vi "GetSetRegister.vi"(7 "Set?":bool, 8 "error in (no error)":errorcluster, 9 "Bytes in":string, 10 "Register Name":string, 11 "Camera in":refnum<class "Camera.lvclass">) -> (0 "error out":errorcluster, 1 "Bytes out":string)   [LabVIEW 2020, in "Camera.lvclass"]
uses:
  Camera.lvclass
  Camera.lvclass/Camera.ctl
  bin/gindustrialcam_32-1.dll
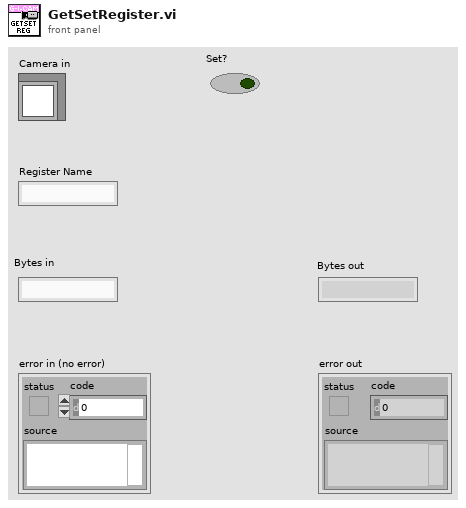
[diagram p1: front panel]
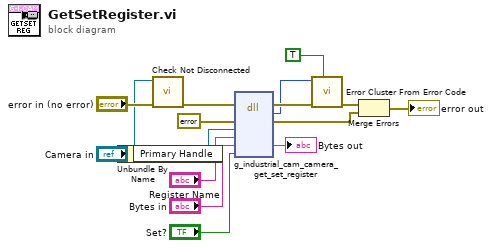
[diagram p0: block diagram]
diagram:
  n1 = Unbundle By Name("Camera in") -> ("Primary Handle"=w5:refnum<data-value>)
  n2 = call "Check Not Disconnected.vi"("error in (no error)"="error in (no error)", "Camera in"="Camera in") -> ("error out"=w2:errorcluster)  [unwired: 9 in]
  n3 = dll-call lib="C:/serenial/lib/g-industrial-camera/LabVIEW/g_industrial_cam/bin/gindustrialcam_*-1.*" fn="g_industrial_cam_camera_get_set_register"(error in=w2, "err"=errorcluster {"status"=FALSE, "code"=0, "source"=""} ("error constant"), "edvr"=w5, "name"="Register Name", "value"="Bytes in", "set"="Set?") -> (error out=w15:errorcluster, "Mg_Error"=w14:i32, "err"=w12:errorcluster, "value"=→"Bytes out":string)  [unwired: 5 in, 1 out]
  n4 = call <vilib>:"Error Cluster From Error Code.vi"("show call chain? (False)"=TRUE, "error in (no error)"=w15, "error code (0)"=w14) -> ("error out"=w13:errorcluster)  [unwired: 6 in]
  n5 = Merge Errors(w13, w12) -> (→"error out":errorcluster)
